vi "process(Server).vi"(8 "error in (no error)":errorcluster, 10 "Sync":refnum<notifier>, 11 "Session in":refnum<class "Session.lvclass">) -> (0 "error out":errorcluster, 3 "Session out":refnum<class "Session.lvclass">)   [LabVIEW 2013, in "MQTT Server.lvlib" / "Session.lvclass"]
uses:
  Session.lvclass
  Control Packets/ControlPacket/ControlPacket.lvclass
  Session.lvclass/Session.ctl
  Connection/TCPConnection.lvclass
panel:
  out "bytes stored":i32
  out "timed out":bool
  out "Numeric 2":i32
  out "Numeric":i32
  out "Last Request":timestamp
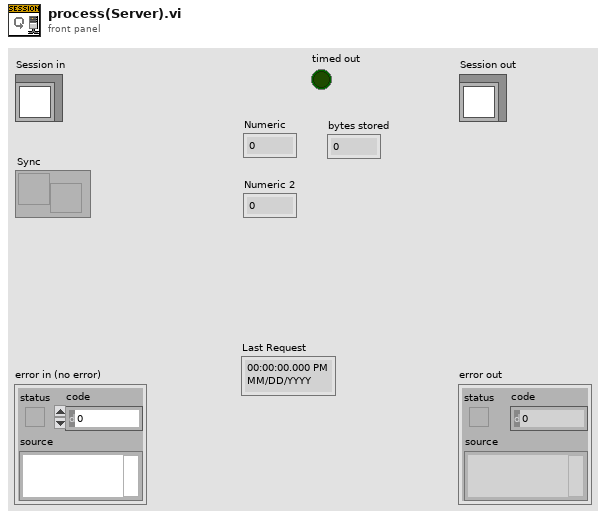
[diagram p1: front panel]
types:
  T1 = enum16{"Standard", "Buffered", "CRLF", "Immediate"}
  T2 = typedef "MQTT Server.lvlib/MQTT_Base.lvclass/Response -- cluster.ctl" = cluster{"Packet":refnum<class "ControlPacket.lvclass">, "Protocol Error":errorcluster, "disconnect session":bool}
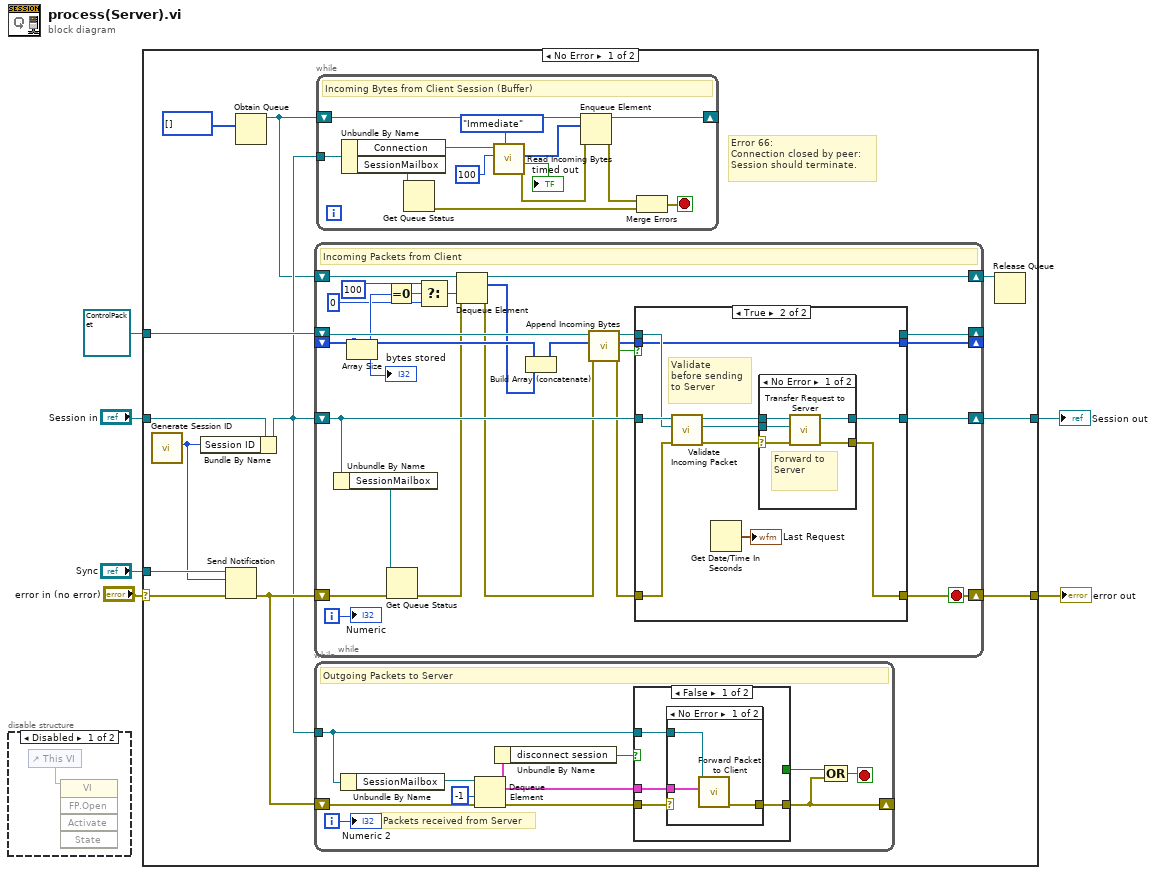
[diagram p0: block diagram]
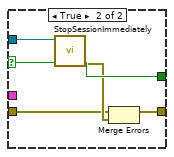
[diagram p4: hidden frame]
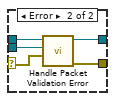
[diagram p6: hidden frame]
diagram:
  n1 = disable-structure shown="Disabled" {
    frame Disabled {
      n2 = control-ref of="This VI"() -> (w7:refnum<vi>)
      n3 = invoke class="VI" method="FP.Open"(reference=w7) -> ()  [unwired: 4 in, 5 out]
    }
    frame Enabled {
    }
  }
  n4 = case shown="No Error" "error in (no error)" {
    selector: "error in (no error)" -> [w14 w107]
    tunnel: [w16 w107] -> w3
    tunnel: [w15 w106] -> w2
    tunnel: "Session in" -> [w18 w106]
    tunnel: refnum<class "ControlPacket.lvclass"> refnum ("Incomplete ControlPacket") -> [w19 _]
    tunnel: "Sync" -> [w17 _]
    frame No Error {
      # "Error 66: \nConnection closed by peer:\nSession should terminate."
      n5 = call "Generate Session ID.vi"() -> ("Session ID"=w12:i32)  [unwired: 11 in]
      n6 = Bundle By Name(cluster=w18, "Session ID"=w12) -> (w11:refnum<class "Session.lvclass">)
      n7 = Send Notification(notification=w12, notifier=w17, error in (no error)=w14) -> (error out=w13:errorcluster)  [unwired: 1 out]
      n8 = Obtain Queue(element data type=u8[] [] ("Bytes")) -> (queue out=w9:refnum<queue>)  [unwired: 4 in, 2 out]
      n9 = while {
        shift-right: [w77] -> w15
        shift-left: w11 -> [w76]
        shift-right: [w71] -> w16
        shift-left: w13 -> [w74]
        shift-right: [w80] -> _
        shift-left: w19 -> [w81]
        shift-right: [w79] -> _
        shift-left: _ -> [w72]
        shift-right: [w64] -> w8
        shift-left: w9 -> [w66]
        i -> [w73]
        stop <- w71 stop-if-true
        # "Incoming Packets from Client"
        n10 = Unbundle By Name(w76) -> ("SessionMailbox"=w75:refnum<queue>)
        n11 = Array Size(array=w72) -> (size(s)=w62:i32)
        "bytes stored" <- w62
        n12 = Equal To 0?(x=w62) -> (x = 0?=w63:bool)
        n13 = Get Queue Status(queue=w75, error in (no error)=w74) -> (error out=w58:errorcluster)  [unwired: 1 in, 7 out]
        n14 = Select(t=100 ("timeout in ms (-1)"), s=w63, f=0 ("timeout in ms (-1)")) -> (s? t:f=w59:i32)
        n15 = Dequeue Element(queue=w66, timeout in ms (-1)=w59, error in (no error)=w58) -> (queue out=w64:refnum<queue>, element=w65:u8[], error out=w57:errorcluster)  [unwired: 1 out]
        n16 = Build Array (concatenate)(w72, w65) -> (w78:u8[])
        n17 = call "Append Incoming Bytes.vi"("error in (no error)"=w57, "Incoming Packets"=w78, "Incomplete ControlPacket"=w81) -> ("error out"=w67:errorcluster, "Complete Packet"=w70:bool, "Remaining Packets"=w68:u8[], "ControlPacket"=w69:refnum<class "ControlPacket.lvclass">)  [unwired: 5 in]
        n18 = case shown="True" w70 {
          tunnel: w69 -> [w85 w92]
          tunnel: [w85 _] -> w80
          tunnel: w68 -> [w84 w86]
          tunnel: [w84 w86] -> w79
          tunnel: [w83 w94] -> w77
          tunnel: w76 -> [w83 w93]
          tunnel: [w82 w87] -> w71
          tunnel: w67 -> [w82 w88]
          frame False {
          }
          frame True {
            # "Validate\nbefore sending\nto Server"
            n19 = call "Validate Incoming Packet.vi"("error in (no error)"=w88, "ControlPacket"=w92, "Session in"=w93) -> ("error out"=w89:errorcluster, "ControlPacket out"=w90:refnum<class "ControlPacket.lvclass">, "Session out"=w91:refnum<class "Session.lvclass">)  [unwired: 6 in]
            n20 = Get Date/Time In Seconds() -> (seconds since 1Jan1904=→"Last Request":timestamp)
            n21 = case shown="No Error" w89 {
              selector: w89 -> [w96 w103]
              tunnel: [w100 w101] -> w94
              tunnel: w91 -> [w99 w105]
              tunnel: w90 -> [w98 w104]
              tunnel: [w97 w102] -> w87
              frame No Error {
                # "Forward to Server"
                n22 = call "Transfer Request to Server.vi"("error in (no error)"=w96, "ServerRequest"=w98, "Session in"=w99) -> ("error out"=w97:errorcluster, "Session out"=w100:refnum<class "Session.lvclass">)  [unwired: 7 in]
              }
              frame Error {
                n23 = call "Handle Packet Validation Error.vi"("Packet Validation Error"=w103, "ControlPacket"=w104, "Session in"=w105) -> ("error out"=w102:errorcluster, "Session out"=w101:refnum<class "Session.lvclass">)  [unwired: 7 in]
              }
            }
          }
        }
        "Numeric" <- w73
      }
      n24 = while {
        tunnel: w11 -> [w39]
        shift-right: [w36] -> _
        shift-left: w13 -> [w40]
        i -> [w33]
        stop <- w35 stop-if-true
        # "Packets received from Server"
        # "Outgoing Packets to Server"
        n25 = Unbundle By Name(w39) -> ("SessionMailbox"=w43:refnum<queue>)
        n26 = Dequeue Element(queue=w43, timeout in ms (-1)=-1, error in (no error)=w40) -> (element=w38:T2, error out=w41:errorcluster)  [unwired: 2 out]
        n27 = Unbundle By Name(w38) -> ("disconnect session"=w37:bool)
        n28 = case shown="False" w37 {
          selector: w37 -> [_ w56]
          tunnel: w41 -> [w47 w53]
          tunnel: [w46 w52] -> w36
          tunnel: w39 -> [w45 w55]
          tunnel: w38 -> [w44 _]
          tunnel: [_ w56] -> w34
          frame False {
            n29 = case shown="No Error" w47 {
              selector: w47 -> [_ w51]
              tunnel: w44 -> [w50 _]
              tunnel: [w49 w51] -> w46
              tunnel: w45 -> [w48 _]
              frame No Error {
                n30 = call "Forward Packet to Client.vi"("Response"=w50, "Session in"=w48) -> ("error out"=w49:errorcluster)  [unwired: 9 in]
              }
              frame Error {
              }
            }
          }
          frame True {
            n31 = call "StopSessionImmediately.vi"("Session in"=w55) -> ("error out"=w54:errorcluster)  [unwired: 9 in, 1 out]
            n32 = Merge Errors(w53, w54) -> (w52:errorcluster)
          }
        }
        n33 = Compound Arithmetic op=OR(w34, w36) -> (w35:bool)
        "Numeric 2" <- w33
      }
      n34 = while {
        tunnel: w11 -> [w32]
        shift-right: [w24] -> _
        shift-left: w9 -> [w25]
        stop <- w26 stop-if-true
        # "Incoming Bytes from Client Session (Buffer)"
        n35 = Unbundle By Name(w32) -> ("Connection"=w29:refnum<class "TCPConnection.lvclass">, "SessionMailbox"=w31:refnum<queue>)
        n36 = Get Queue Status(queue=w31) -> (error out=w27:errorcluster)  [unwired: 2 in, 7 out]
        n37 = call "Read Incoming Bytes.vi"("mode (standard)"=T1."Immediate", "bytes to read (100)"=100, "TCPConnection in"=w29) -> ("error out"=w22:errorcluster, "timed out"=→"timed out":bool, "Bytes"=w23:u8[])  [unwired: 5 in, 1 out]
        n38 = Enqueue Element(queue=w25, element=w23, error in (no error)=w22) -> (queue out=w24:refnum<queue>, error out=w21:errorcluster)  [unwired: 1 in, 1 out]
        n39 = Merge Errors(w21, w27) -> (w26:errorcluster)
      }
      n40 = Release Queue(queue=w8) -> ()  [unwired: 2 in, 3 out]
    }
    frame Error {
    }
  }
  "error out" <- w3
  "Session out" <- w2
